vi "LVITX XY Plot Commands W2D.vi"(0 "wavenames":string[](array[string])=["'IV0_summ.itx.0003'[0][0]", "'IV0_summ.itx.0003'[0][1]", "'IV0_summ.itx.0003'[0][2]", "'IV0_summ.itx.0003'[0][3]", "'IV0_summ.itx.0003'[0][4]", "'IV0_summ.itx.0003'[0][5]", "'IV0_summ.itx.0003'[0][6]", "'IV0_summ.itx.0003'[0][7]", "'IV0_summ.itx.0003'[0][8]", "'IV0_summ.itx.0003'[0][9]", "'IV0_summ.itx.0003'[0][10]", "'IV0_summ.itx.0003'[0][11]", "'IV0_summ.itx.0003'[0][12]", "'IV0_summ.itx.0003'[0][13]", "'IV0_summ.itx.0003'[0][14]", "'IV0_summ.itx.0003'[0][15]", "'IV0_summ.itx.0003'[0][16]", "'IV0_summ.itx.0003'[0][17]", "'IV0_summ.itx.0003'[0][18]", "'IV0_summ.itx.0003'[0][19]", "'IV0_summ.itx.0003'[0][20]"], 1 "X label":string="energy (eV)", 2 "Y label":string="amplitude (arb)", 3 "input string":string="Display #wave# vs '#waveX#'\nAppendToGraph #wave# vs '#waveX#'\nLabel bottom \"#labelX#\"\nLabel left \"#labelY#\"\nModifyGraph rgb(#wave#)=(#r#,#g#,#b#)\nLegend/C/N=text0\nModifyGraph mirror=1", 4 "X wave":string="x_") -> (5 "result string":string="Display 'IV0_summ.itx.0003'[0][0] vs 'x_'\nAppendToGraph 'IV0_summ.itx.0003'[0][1] vs 'x_'\nAppendToGraph 'IV0_summ.itx.0003'[0][2] vs 'x_'\nAppendToGraph 'IV0_summ.itx.0003'[0][3] vs 'x_'\nAppendToGraph 'IV0_summ.itx.0003'[0][4] vs 'x_'\nAppendToGraph 'IV0_summ.itx.0003'[0][5] vs 'x_'\nAppendToGraph 'IV0_summ.itx.0003'[0][6] vs 'x_'\nAppendToGraph 'IV0_summ.itx.0003'[0][7] vs 'x_'\nAppendToGraph 'IV0_summ.itx.0003'[0][8] vs 'x_'\nAppendToGraph 'IV0_summ.itx.0003'[0][9] vs 'x_'\nAppendToGraph 'IV0_summ.itx.0003'[0][10] vs 'x_'\nAppendToGraph 'IV0_summ.itx.0003'[0][11] vs 'x_'\nAppendToGraph 'IV0_summ.itx.0003'[0][12] vs 'x_'\nAppendToGraph 'IV0_summ.itx.0003'[0][13] vs 'x_'\nAppendToGraph 'IV0_summ.itx.0003'[0][14] vs 'x_'\nAppendToGraph 'IV0_summ.itx.0003'[0][15] vs 'x_'\nAppendToGraph 'IV0_summ.itx.0003'[0][16] vs 'x_'\nAppendToGraph 'IV0_summ.itx.0003'[0][17] vs 'x_'\nAppendToGraph 'IV0_summ.itx.0003'[0][18] vs 'x_'\nAppendToGraph 'IV0_summ.itx.0003'[0][19] vs 'x_'\nAppendToGraph 'IV0_summ.itx.0003'[0][20] vs 'x_'\nLabel bottom \"energy (eV)\"\nLabel left \"amplitude (arb)\"\nModifyGraph rgb('IV0_summ.itx.0003'[0][0])=(65280,0,0)\nModifyGraph rgb('IV0_summ.itx.0003'[0][1])=(65280,16896,0)\nModifyGraph rgb('IV0_summ.itx.0003'[0][2])=(65280,33792,0)\nModifyGraph rgb('IV0_summ.itx.0003'[0][3])=(65280,50688,0)\nModifyGraph rgb('IV0_summ.itx.0003'[0][4])=(63488,65280,0)\nModifyGraph rgb('IV0_summ.itx.0003'[0][5])=(46592,65280,0)\nModifyGraph rgb('IV0_summ.itx.0003'[0][6])=(29696,65280,0)\nModifyGraph rgb('IV0_summ.itx.0003'[0][7])=(12800,65280,0)\nModifyGraph rgb('IV0_summ.itx.0003'[0][8])=(0,65280,4096)\nModifyGraph rgb('IV0_summ.itx.0003'[0][9])=(0,65280,20992)\nModifyGraph rgb('IV0_summ.itx.0003'[0][10])=(0,65280,37888)\nModifyGraph rgb('IV0_summ.itx.0003'[0][11])=(0,65280,53248)\nModifyGraph rgb('IV0_summ.itx.0003'[0][12])=(0,60928,65280)\nModifyGraph rgb('IV0_summ.itx.0003'[0][13])=(0,44032,65280)\nModifyGraph rgb('IV0_summ.itx.0003'[0][14])=(0,27136,65280)\nModifyGraph rgb('IV0_summ.itx.0003'[0][15])=(0,10240,65280)\nModifyGraph rgb('IV0_summ.itx.0003'[0][16])=(6656,0,65280)\nModifyGraph rgb('IV0_summ.itx.0003'[0][17])=(23552,0,65280)\nModifyGraph rgb('IV0_summ.itx.0003'[0][18])=(40448,0,65280)\nModifyGraph rgb('IV0_summ.itx.0003'[0][19])=(57344,0,65280)\nModifyGraph rgb('IV0_summ.itx.0003'[0][20])=(65280,0,56832)\nLegend/C/N=text0")   [LabVIEW 2011]
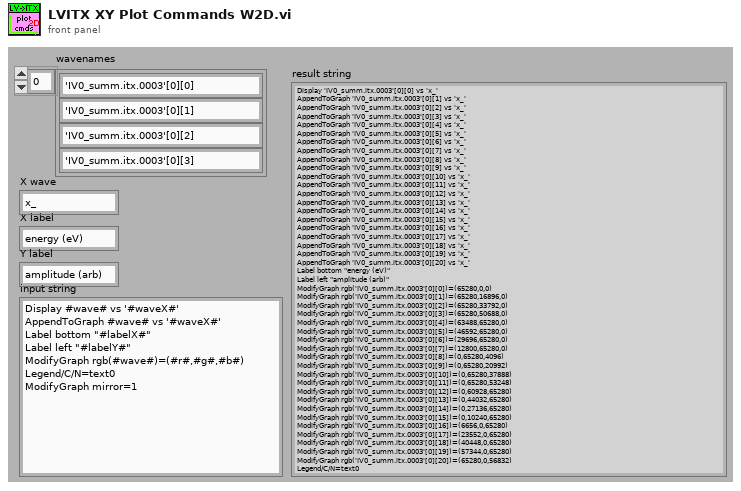
[diagram p1: front panel]
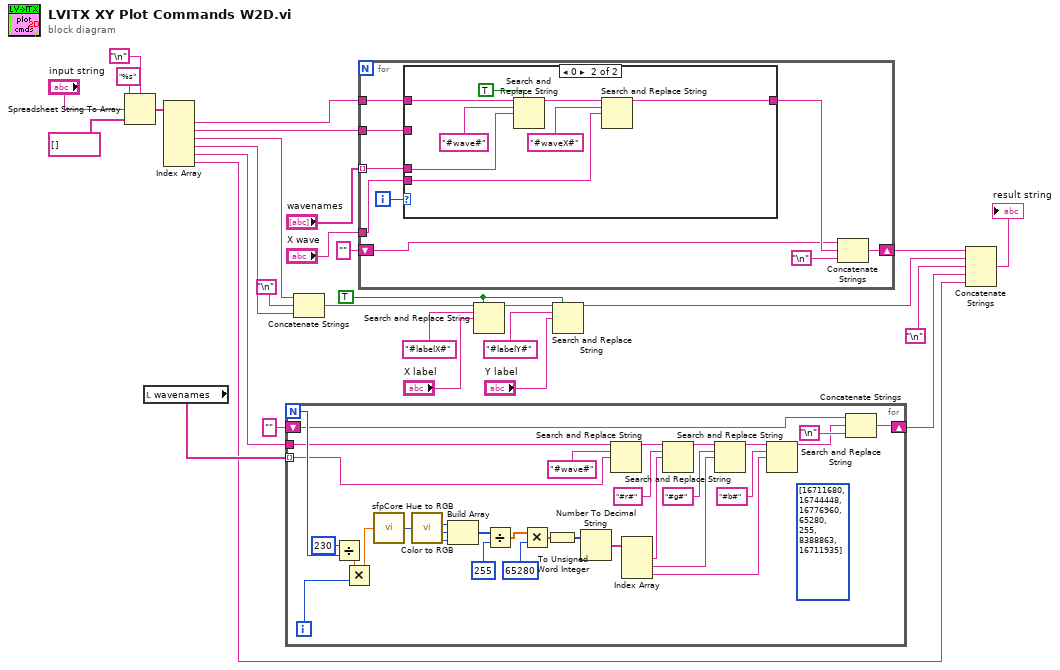
[diagram p0: block diagram]
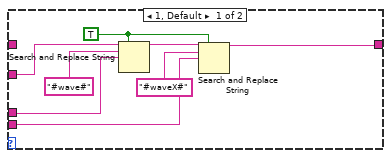
[diagram p2: hidden frame]
diagram:
  w11 = TRUE ("replace all? (F)")
  n1 = Spreadsheet String To Array(delimiter (Tab)="\n", format string="%s", spreadsheet string="input string", array type (2D Dbl)=string[] []) -> (array=w20:string[])
  n2 = local read "wavenames"() -> (w9:string[])
  n3 = Index Array(array=w20) -> (element #1=w19:string, element #2=w18:string, element #3=w1:string, element #4=w2:string, element #5=w3:string, element #6=w4:string)  [unwired: 6 in]
  n4 = for {
    N -> [w50]
    tunnel: w3 -> [w45]
    tunnel: w9 -> [w38] mode=indexing
    shift-right: [w41] -> w8
    shift-left: "" -> [w40]
    i -> [w49]
    (unwired) u32[] [16711680, 16744448, 16776960, 65280, 255, 8388863, 16711935]
    n5 = Divide(x=230, y=w50) -> (x/y=w52:dbl)
    n6 = Multiply(x=w52, y=w49) -> (x*y=w48:dbl)
    n7 = call <userlib>:"sfpCore Hue to RGB.vi"("hue value"=w48) -> ("output color"=w54:u32)
    n8 = call <vilib>:"Color to RGB.vi"("Color"=w54) -> ("R"=w59:u8, "G"=w60:u8, "B"=w61:u8)  [unwired: 1 out]
    n9 = Build Array(w59, w60, w61) -> (w58:u8[])
    n10 = Divide(x=w58, y=255) -> (x/y=w53:dbl[])
    n11 = Multiply(x=w53, y=65280) -> (x*y=w55:dbl[])
    n12 = To Unsigned Word Integer(number=w55) -> (unsigned 16bit integer=w47:u16[])
    n13 = Number To Decimal String(number=w47) -> (decimal integer string=w33:string[])  [unwired: 1 out]
    n14 = Search and Replace String(input string=w45, search string="#wave#", replace string=w38) -> (result string=w46:string)  [unwired: 1 in, 7 out]
    n15 = Index Array(array=w33) -> (element #1=w32:string, element #2=w31:string, element #3=w30:string)  [unwired: 3 in]
    n16 = Search and Replace String(input string=w46, search string="#r#", replace string=w32) -> (result string=w44:string)  [unwired: 1 in, 7 out]
    n17 = Search and Replace String(input string=w44, search string="#g#", replace string=w31) -> (result string=w43:string)  [unwired: 1 in, 7 out]
    n18 = Search and Replace String(input string=w43, search string="#b#", replace string=w30) -> (result string=w37:string)  [unwired: 1 in, 7 out]
    n19 = Concatenate Strings(w40, w37, "\n") -> (w41:string)
  }
  n20 = Concatenate Strings(w1, "\n", w2) -> (w16:string)
  n21 = for {
    tunnel: "wavenames" -> [w68] mode=indexing
    tunnel: w19 -> [w70]
    tunnel: w18 -> [w69]
    shift-right: [w66] -> w24
    shift-left: "" -> [w63]
    tunnel: "X wave" -> [w62]
    i -> [w67]
    n22 = case shown="0" w67 {
      tunnel: w70 -> [_ w84]
      tunnel: w69 -> [w76 _]
      tunnel: w68 -> [w77 w85]
      tunnel: [w72 w81] -> w65
      tunnel: w62 -> [w73 w79]
      frame 1, Default {
        w71 = TRUE ("replace all? (F)")
        n23 = Search and Replace String(replace all?=w71, input string=w76, search string="#wave#", replace string=w77) -> (result string=w75:string)  [unwired: 1 in, 6 out]
        n24 = Search and Replace String(replace all?=w71, input string=w75, search string="#waveX#", replace string=w73) -> (result string=w72:string)  [unwired: 1 in, 6 out]
      }
      frame 0 {
        n25 = Search and Replace String(replace all?=TRUE ("replace all? (F)"), input string=w84, search string="#wave#", replace string=w85) -> (result string=w82:string)  [unwired: 1 in, 6 out]
        n26 = Search and Replace String(input string=w82, search string="#waveX#", replace string=w79) -> (result string=w81:string)  [unwired: 1 in, 7 out]
      }
    }
    n27 = Concatenate Strings(w63, w65, "\n") -> (w66:string)
  }
  n28 = Search and Replace String(replace all?=w11, input string=w16, search string="#labelX#", replace string="X label") -> (result string=w14:string)  [unwired: 1 in, 6 out]
  n29 = Search and Replace String(replace all?=w11, input string=w14, search string="#labelY#", replace string="Y label") -> (result string=w6:string)  [unwired: 1 in, 6 out]
  n30 = Concatenate Strings(w24, w6, "\n", w8, w4) -> (→"result string":string)
